vi "Dashboard Main.vi"() -> ()   [LabVIEW 2012]
uses:
  <vilib>/event_ctls.llb/eventvkey.ctl
  <vilib>/Utility/miscctls.llb/LVPointTypeDef.ctl
  <vilib>/Utility/config.llb/Read Key (String).vi
  <vilib>/Utility/config.llb/Read Key (I32).vi
  <vilib>/Utility/config.llb/Write Key (String).vi
  <vilib>/Utility/config.llb/Write Key (I32).vi
  <vilib>/Utility/config.llb/NI_LVConfig.lvlib
panel:
  out "Battery Value":dbl(slide) scale=0.0..14.0 scale format="%#_2e"
  out "Battery":sgl(graph)
  in  "Camera Settings":T1={"Frate Rate"=30, "Compression"=30, "Size"=0} {"Frate Rate" scale=1.0..30.0; "Size" items=["640x480", "320x240", "160x120"]}
  out "Mode":T2(ring)=enum.""
  out "Camera IP":string="10.16.76.11"
  out "JS1 Z":dbl(slide) scale=-1.0..1.0 scale format="%#_2e"
  out "JS2 Z":dbl(slide) scale=-1.0..1.0 scale format="%#_2e"
  out "Joystick 1":cluster{"X":dbl, "Y":dbl}[](graph)
  out "Joystick 2":cluster{"X":dbl, "Y":dbl}[](graph)
  out "JS Buttons 1":T3
  out "JS Buttons 2":T3
  out "MotorSlide4":dbl(slide) scale=-1.0..1.0 scale format="%#_2e"
  out "MotorSlide3":dbl(slide) scale=-1.0..1.0 scale format="%#_2e"
  out "MotorSlide2":dbl(slide) scale=-1.0..1.0 scale format="%#_2e"
  in  "MotorName3":string="Front Left"
  in  "MotorName4":string="Front Right"
  in  "MotorName1":string="Rear Left"
  in  "MotorName2":string="Rear Right"
  out "MotorChart4":dbl(graph)
  out "MotorChart3":dbl(graph)
  out "MotorChart2":dbl(graph)
  out "MotorSlide1":dbl(slide) scale=-1.0..1.0 scale format="%#_2e"
  out "MotorChart1":dbl(graph)
  out "Robot IP":string="0.0.0.0"
  in  "Dashboard Tab":enum32{"Operation", "Test", "Checklist"}(tab)
  out "Dashboard Code Verzion":string
  out "Robot Code Verzion":string
  out "Gyro":dbl
  out "Encoder Average":dbl
  out "Right Encoder":dbl
  out "Left Encoder":dbl
  out "Vision Angle":dbl
  out "Wheel Speed":dbl
  in  "Process Vision":bool=TRUE
  in  "Slider":dbl(slide) scale=0.0..100.0 scale format="%#_3g"
  in  "On/Off":bool caption="Solenoid"
  in  "Test Name":u16(ring) items=["Select the test to run...", "Example Test", "-------------------------------", "List of tests is built in robot code.", "Replace with your own automated tests."]
  in  "Test Tree":string(tree)
  in  "Motor":cluster{"Value":dbl, "Enable":bool} {"Value" scale=-1.0..1.0 scale format="%#_3g"}
  out "Progress":T4 {"Test Progress" scale=0.0..100.0}
  in  "Rev/Fwd":cluster{"Forward":bool, "Reverse":bool}
  in  "Ring":u16(ring) items=["Auto", "Fixed indoor", "Fixed outdoor 1", "Fixed outdoor 2", "Fixed fluorescent 1", "Fixed fluorescent 2", "Hold current"]
  in  "Listbox":i32(listbox)
  in  "Viewer":T5(tab)
  out "Mbps":dbl format="%#.1g"
  in  "Enable":bool=TRUE
  in  "DB Camera Config":bool
  out "Mbps":bool
  out "fps":dbl format="%#.1g"
  out "Image Error Message":string="Timeout in Camera Communications"
  out "Camera Image":T6(plugin-control)
  out "Buttons 1":cluster{"1":bool, "2":bool, "3":bool}
  out "Kinect 1":cluster{"X":dbl, "Y":dbl, "Z":dbl} {"X" scale=1.0..-1.0; "Y" scale=1.0..-1.0; "Z" scale=1.0..-1.0}
  out "Buttons 2":cluster{"1":bool, "2":bool, "3":bool}
  out "Kinect 2":cluster{"X":dbl, "Y":dbl, "Z":dbl} {"X" scale=1.0..-1.0; "Y" scale=1.0..-1.0; "Z" scale=1.0..-1.0}
  out "Version":string
  out "Skeleton Picture":picture
  out "Players":i8
  out "Tree":string(tree)
  # "Drive & Motors"
  # "Robot IP:"
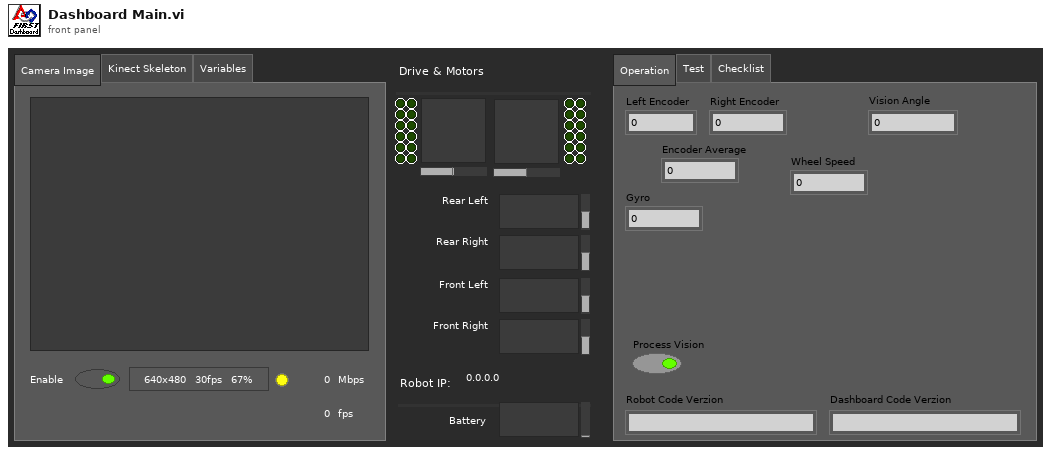
[diagram p1: front panel]
types:
  T1 = cluster{"Frate Rate":i32, "Compression":i32, "Size":u16}
  T2 = enum8{"Tele-Op Disabled", "Tele-Op Enabled", "Auto Disabled", "Auto Enabled", "Test Disabled", "Test Enabled", ""}
  T3 = cluster{bool, bool, bool, bool, bool, bool, bool, bool, bool, bool, bool, bool}
  T4 = cluster{"Test Progress":u8, "Test Progress Text":string}
  T5 = enum32{"Camera Image", "Kinect Skeleton", "Variables"}
  T6 = typedef "IMAQ Image.ctl" = refnum<image>
  T7 = typedef "Image Type" = u32
  T8 = cluster{"Competition mode":bool, "Robot Link":bool, "Autonomous":bool, "Enabled":bool, "E-Stop":bool, "Simulated":bool, "TestMode":bool, "Docked Window":bool}
  T9 = cluster{"Boolean Array[0]":bool, "Boolean Array[1]":bool, "Boolean Array[2]":bool, "Boolean Array[3]":bool, "Boolean Array[4]":bool, "Boolean Array[5]":bool, "Boolean Array[6]":bool, "Boolean Array[7]":bool, "Boolean Array[8]":bool, "Boolean Array[9]":bool, "Boolean Array[10]":bool, "Boolean Array[11]":bool}
  T10 = typedef "LVPointTypeDef.ctl" = cluster{"Horizontal":i16, "Vertical":i16}
  T11 = typedef "LVRectTypeDef.ctl" = cluster{"Left":i16, "Top":i16, "Right":i16, "Bottom":i16}
  T12 = typedef "LVBoundsTypeDef.ctl" = cluster{"Width":u32, "Height":u32}
  T13 = typedef "SkeletonTrackState.ctl" = enum32{"NotTracked", "PositionOnly", "Tracked"}
  T14 = cluster{"TrackingState":u8[], "Position":cluster{"x":sgl, "y":sgl, "z":sgl}, cluster{"x":sgl, "y":sgl, "z":sgl, sgl}[], "TrackState":T13}
  T15 = cluster{cluster{"ScaledToPercentRange":dbl, "ScaledToPercentRange":dbl, "ScaledToPercentRange":dbl}, cluster{bool, bool, bool}}[]
  T16 = cluster{cluster{"ScaledToPercentRange":dbl, "ScaledToPercentRange":dbl, "ScaledToPercentRange":dbl}, cluster{bool, bool, bool}}
  T17 = cluster{"ScaledToPercentRange":dbl, "ScaledToPercentRange":dbl, "ScaledToPercentRange":dbl}
  T18 = typedef "NI_LVConfig.lvlib/Config Data RefNum.ctl" = refnum<k1>
  T19 = typedef "eventvkey.ctl" = enum16{"ASCII", "Enter", "Return", "Shift", "Ctrl", "Alt", "Cmd", "Opt", "Caps", "NumLock", "Clear", "Break", "Up", "Down", "Left", "Right", "Insert", "Delete", "Home", "End", "PageUp", "PageDown", "Escape", "Help", "Pause", "ScrollLock", "F1", "F2", "F3", "F4", "F5", "F6", "F7", "F8", "F9", "F10", "F11", "F12", "F13", "F14", "F15", "F16", "F17", "F18", "F19", "F20", "F21", "F22", "F23", "F24", "Play", "VolumeUp", "VolumeDown", "Mute", "Two Byte Char"}
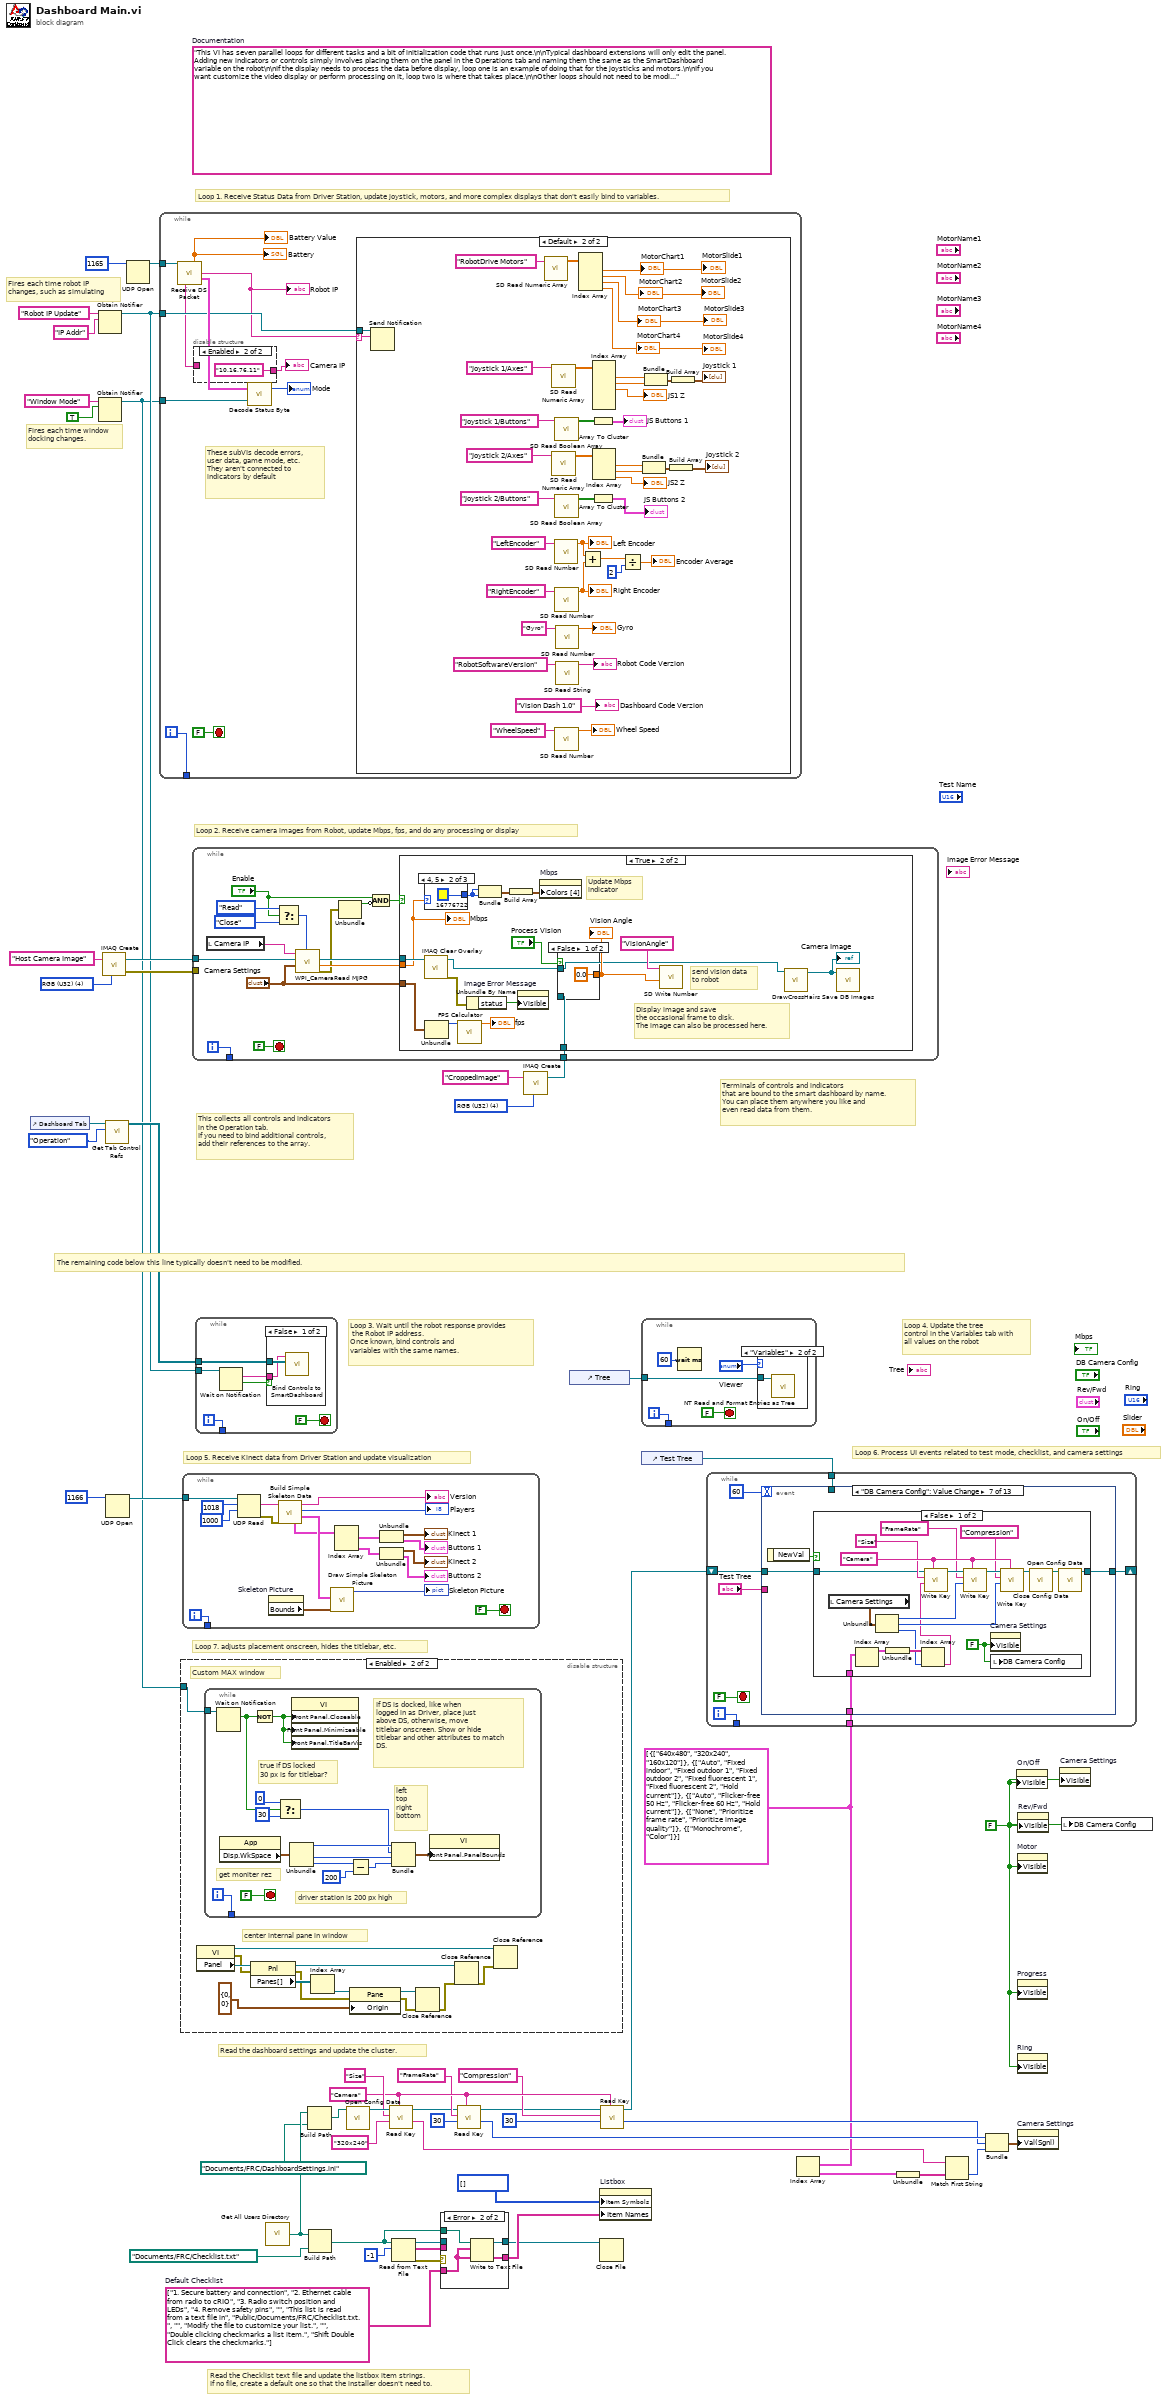
[diagram p0: block diagram]
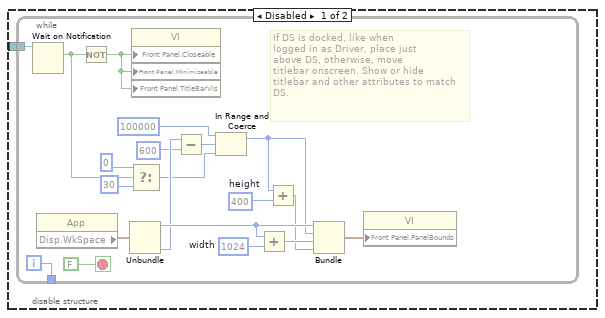
[diagram p2: hidden frame]
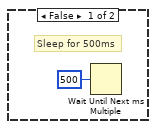
[diagram p4: hidden frame]
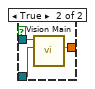
[diagram p5: hidden frame]
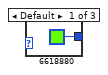
[diagram p6: hidden frame]
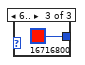
[diagram p7: hidden frame]
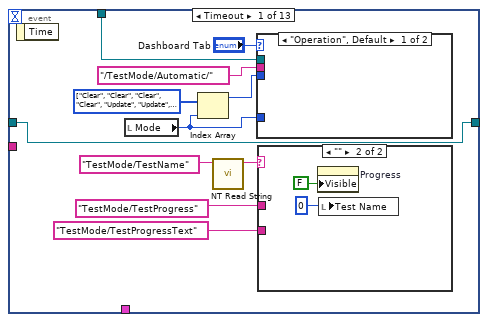
[diagram p9: hidden frame]
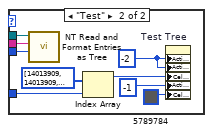
[diagram p10: hidden frame]
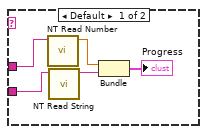
[diagram p11: hidden frame]
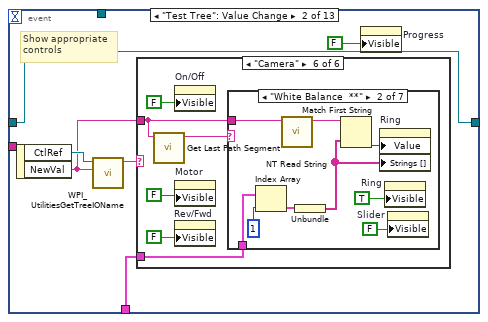
[diagram p12: hidden frame]
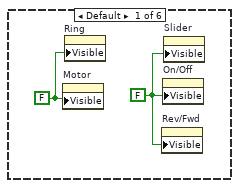
[diagram p13: hidden frame]
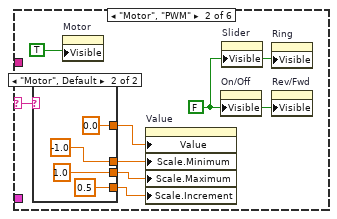
[diagram p14: hidden frame]
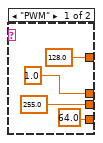
[diagram p15: hidden frame]
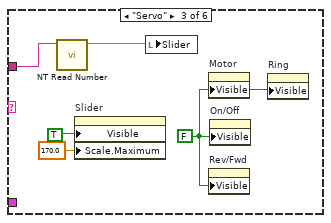
[diagram p16: hidden frame]
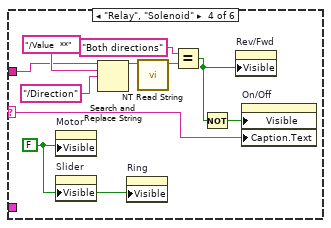
[diagram p17: hidden frame]
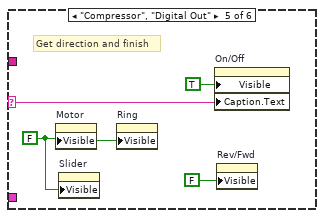
[diagram p18: hidden frame]
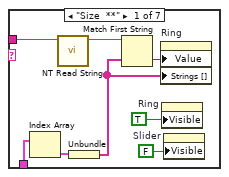
[diagram p19: hidden frame]
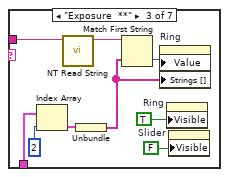
[diagram p20: hidden frame]
diagram:
  w2 = T7 4 items=["Grayscale (U8)", "Grayscale (I16)", "Grayscale (SGL)", "Complex (CSG)", "RGB (U32)", "HSL (U32)", "RGB (U64)", "Grayscale (U16)"] ("Image Type")
  w24 = "Camera"
  w16 = cluster{string[]}[] [{["640x480", "320x240", "160x120"]}, {["Auto", "Fixed indoor", "Fixed outdoor 1", "Fixed outdoor 2", "Fixed fluorescent 1", "Fixed fluorescent 2", "Hold current"]}, {["Auto", "Flicker-free 50 Hz", "Flicker-free 60 Hz", "Hold current"]}, {["None", "Prioritize frame rate", "Prioritize image quality"]}, {["Monochrome", "Color"]}]
  w32 = string[] ["1. Secure battery and connection", "2. Ethernet cable from radio to cRIO", "3. Radio switch position and LEDs", "4. Remove safety pins", "", "This list is read from a text file in", "Public/Documents/FRC/Checklist.txt.", "", "Modify the file to customize your list.", "", "Double clicking checkmarks a list item.", "Shift Double Click clears the checkmarks."]  # Default Checklist
  w30 = FALSE ("Visible")
  (unwired) "This VI has seven parallel loops for different tasks and a bit of initialization code that runs just once.\n\nTypical dashboard extensions will only edit the panel. Adding new indicators or controls simply involves placing them on the panel in the Operations tab and naming them the same as the SmartDashboard variable on the robot\n\nIf the display needs to process the data before display, loop one is an example of doing that for the joysticks and motors.\n\nIf you want customize the video display or perform processing on it, loop two is where that takes place.\n\nOther loops should not need to be modified. They are pretty standard, and document the task they perform."  # Documentation
  w53 = T7 4 items=["Grayscale (U8)", "Grayscale (I16)", "Grayscale (SGL)", "Complex (CSG)", "RGB (U32)", "HSL (U32)", "RGB (U64)"] ("Image Type")
  # "Fires each time robot IP\nchanges, such as simulating"
  # "Fires each time window\ndocking changes."
  # "Read the Checklist text file and update the listbox item strings.\nIf no file, create a default one so that the installer doesn't need to."
  # "This collects all controls and indicators\nin the Operation tab.\nIf you need to bind additional controls,\nadd their references to the array."
  # "The remaining code below this line typically doesn't need to be modified."
  # "Loop 6. Process UI events related to test mode, checklist, and camera settings"
  # "Read the dashboard settings and update the cluster."
  # "Terminals of controls and indicators\nthat are bound to the smart dashboard by name.\nYou can place them anywhere you like and\neven read data from them."
  # "Loop 4. Update the tree\ncontrol in the Variables tab with\nall values on the robot"
  # "Loop 3. Wait until the robot response provides\n the Robot IP address.\nOnce known, bind controls and\nvariables with the same names."
  # "Loop 5. Receive Kinect data from Driver Station and update visualization"
  # "Loop 7. adjusts placement onscreen, hides the titlebar, etc."
  # "Loop 1. Receive Status Data from Driver Station, update joystick, motors, and more complex displays that don't easily bind to variables."
  # "Loop 2. Receive camera images from Robot, update Mbps, fps, and do any processing or display"
  n1 = control-ref of="Dashboard Tab"() -> (w46:refnum<vi>)
  n2 = Obtain Notifier(name (unnamed)="Robot IP Update", notification data type="IP Addr" ("name (unnamed)")) -> (notifier out=w43:refnum<notifier>)  [unwired: 2 in, 2 out]
  n3 = Obtain Notifier(name (unnamed)="Window Mode", notification data type=TRUE) -> (notifier out=w36:refnum<notifier>)  [unwired: 2 in, 2 out]
  n4 = call "IMAQ Create"("Image Name"="Host Camera Image", "Image Type"=w53) -> ("New Image"=w51:T6, "error out"=w50:errorcluster)  [unwired: 2 in, 1 out]
  n5 = call <vilib>:"Get Tab Control Refs.vi"("Page Index"=enum32{"Operation", "Test"}."Operation" ("Dashboard Tab"), "TabControl in"=w46) -> ("ControlsOnPage"=w47:refnum<vi>[])  [unwired: 9 in]
  n6 = UDP Open(11:u16 1166 ("port")) -> (port=w48:refnum<k16>)  [unwired: 2 in, 4 out]
  n7 = UDP Open(11:u16 1165 ("port")) -> (port=w54:refnum<k16>)  [unwired: 2 in, 4 out]
  n8 = while {
    tunnel: w54 -> [w64]
    tunnel: w43 -> [w59]
    tunnel: w36 -> [w62]
    tunnel: [w60] -> _
    i -> [w60]
    stop <- FALSE stop-if-true
    # "These subVIs decode errors, user data, game mode, etc.\nThey aren't connected to indicators by default"
    n9 = call "Receive DS Packet.vi"("Recv Socket"=w64) -> ("Battery"=→"Battery" →"Battery Value":sgl, "Robot IP Address"=w58:string, "Status"=w65:T8, "Camera IP Address"=w56:string)  [unwired: 1 in, 10 out]
    "Robot IP" <- w58
    n10 = disable-structure shown="Enabled" {
      disable-tunnel: [w67 "10.16.76.11" ("Camera IP")] -> w57
      disable-tunnel: w56 -> [w67 _]
      frame Disabled {
      }
      frame Enabled {
      }
    }
    "Camera IP" <- w57
    n11 = call "Decode Status Byte.vi"("Window Mode Notifier"=w62, "Status"=w65) -> ("Mode"=→"Mode":T2)  [unwired: 1 out]
    n12 = case shown="Default" w58 {
      selector: w58 -> [_ w83]
      tunnel: w59 -> [_ w84]
      frame "0.0.0.0" {
        # "Robot not responding, don't poll the variables"
      }
      frame Default {
        n13 = Send Notification(notification=w83, notifier=w84) -> ()  [unwired: 1 in, 2 out]
        n14 = call <vilib>:"SD Read Numeric Array.vi"("Name"="RobotDrive Motors") -> ("Numeric Array"=w107:dbl[])  [unwired: 8 in, 2 out]
        n15 = call <vilib>:"SD Read Numeric Array.vi"("Name"="Joystick 1/Axes") -> ("Numeric Array"=w100:dbl[])  [unwired: 8 in, 2 out]
        n16 = call <vilib>:"SD Read Numeric Array.vi"("Name"="Joystick 2/Axes") -> ("Numeric Array"=w94:dbl[])  [unwired: 8 in, 2 out]
        n17 = call <vilib>:"SD Read Number.vi"("Name"="LeftEncoder") -> ("Numeric"=w79:dbl)  [unwired: 8 in, 2 out]
        "Left Encoder" <- w79
        n18 = call <vilib>:"SD Read Boolean Array.vi"("Name"="Joystick 1/Buttons") -> ("Boolean Array"=w102:bool[])  [unwired: 8 in, 2 out]
        n19 = call <vilib>:"SD Read Boolean Array.vi"("Name"="Joystick 2/Buttons") -> ("Boolean Array"=w93:bool[])  [unwired: 8 in, 2 out]
        n20 = call <vilib>:"SD Read Number.vi"("Name"="RightEncoder") -> ("Numeric"=w78:dbl)  [unwired: 8 in, 2 out]
        "Right Encoder" <- w78
        n21 = call <vilib>:"SD Read Number.vi"("Name"="WheelSpeed") -> ("Numeric"=→"Wheel Speed":dbl)  [unwired: 8 in, 2 out]
        n22 = call <vilib>:"SD Read Number.vi"("Name"="Gyro") -> ("Numeric"=→"Gyro":dbl)  [unwired: 8 in, 2 out]
        n23 = call <vilib>:"SD Read String.vi"("Name"="RobotSoftwareVersion") -> ("String"=→"Robot Code Verzion":string)  [unwired: 8 in, 2 out]
        n24 = Index Array(array=w107) -> (element #1=→"MotorChart1" →"MotorSlide1":dbl, element #2=→"MotorSlide2" →"MotorChart2":dbl, element #3=→"MotorChart3" →"MotorSlide3":dbl, element #4=→"MotorChart4" →"MotorSlide4":dbl)  [unwired: 4 in]
        n25 = Add(x=w79, y=w78) -> (x+y=w76:dbl)
        n26 = Array To Cluster(array=w102) -> (cluster=→"JS Buttons 1":T9)
        n27 = Array To Cluster(array=w93) -> (cluster=→"JS Buttons 2":T9)
        n28 = Index Array(array=w100) -> (element #1=w97:dbl, element #2=w98:dbl, element #3=→"JS1 Z":dbl)  [unwired: 6 in, 3 out]
        n29 = Index Array(array=w94) -> (element #1=w89:dbl, element #2=w88:dbl, element #3=→"JS2 Z":dbl)  [unwired: 3 in]
        n30 = Divide(x=w76, y=2) -> (x/y=→"Encoder Average":dbl)
        n31 = Bundle("Numeric"=w89, "Numeric"=w88) -> (w90:cluster{"Numeric":dbl, "Numeric":dbl})  [unwired: 1 in]
        n32 = Bundle("Numeric"=w97, "Numeric"=w98) -> (w96:cluster{"Numeric":dbl, "Numeric":dbl})  [unwired: 1 in]
        n33 = Build Array(w90) -> (→"Joystick 2":cluster{"Numeric":dbl, "Numeric":dbl}[])
        n34 = Build Array(w96) -> (→"Joystick 1":cluster{"Numeric":dbl, "Numeric":dbl}[])
        "Dashboard Code Verzion" <- "Vision Dash 1.0" ("Dashboard Code Verzion")
      }
    }
  }
  n35 = disable-structure shown="Enabled" {
    disable-tunnel: w36 -> [w111 w144]
    frame Disabled {
      n36 = while {
        tunnel: w111 -> [w130]
        tunnel: [w128] -> _
        i -> [w128]
        stop <- FALSE stop-if-true
        w120 = 1024  # width
        w123 = 400  # height
        # "If DS is docked, like when\nlogged in as Driver, place just\nabove DS, otherwise, move\ntitlebar onscreen. Show or hide\ntitlebar and other attributes to match\nDS."
        n37 = Wait on Notification(notifier=w130) -> (notification=w115:bool)  [unwired: 3 in, 3 out]
        n38 = property class="App"() -> ("Disp.WkSpace"=w126:T11)  [unwired: 2 in, 2 out]
        n39 = Not(x=w115) -> (.not. x?=w129:bool)
        n40 = Unbundle(w126) -> ("Left"=w124:i16, "Bottom"=w121:i16)  [unwired: 2 out]
        n41 = Select(t=0, s=w115, f=30) -> (s? t:f=w114:i32)
        n42 = property class="VI"("Front Panel.Closeable"=w129, "Front Panel.Minimizeable"=w129, "Front Panel.TitleBarVis"=w129) -> ()  [unwired: 2 in, 2 out]
        n43 = Subtract(x=w121, y=600) -> (x-y=w118:i32)
        n44 = In Range and Coerce(upper limit=100000, x=w118, lower limit=w114) -> (coerced(x)=w112:i32)  [unwired: 1 out]
        n45 = Add(x=w124, y=w120) -> (x+y=w125:i32)
        n46 = Add(x=w112, y=w123) -> (x+y=w122:i32)
        n47 = Bundle("Left"=w124, w112, w125, w122) -> (w127:cluster{"Left":i16, i32, i32, i32})  [unwired: 1 out]
        n48 = property class="VI"("Front Panel.PanelBounds"=w127) -> ()  [unwired: 2 in, 2 out]
      }
    }
    frame Enabled {
      # "center internal pane in window"
      # "Custom MAX window"
      n49 = property class="VI"() -> (reference out=w137:refnum<vi>, error out=w136:errorcluster, "Panel"=w143:refnum<vi>)  [unwired: 2 in]
      n50 = while {
        tunnel: w144 -> [w158]
        tunnel: [w156] -> _
        i -> [w156]
        stop <- FALSE stop-if-true
        # "driver station is 200 px high"
        # "true if DS locked\n30 px is for titlebar?"
        # "left\ntop\nright\nbottom"
        # "get moniter rez"
        # "If DS is docked, like when\nlogged in as Driver, place just\nabove DS, otherwise, move\ntitlebar onscreen. Show or hide\ntitlebar and other attributes to match\nDS."
        n51 = Wait on Notification(notifier=w158) -> (notification=w150:bool)  [unwired: 3 in, 3 out]
        n52 = property class="App"() -> ("Disp.WkSpace"=w154:T11)  [unwired: 2 in, 2 out]
        n53 = Not(x=w150) -> (.not. x?=w157:bool)
        n54 = Select(t=0, s=w150, f=30) -> (s? t:f=w148:i32)
        n55 = Unbundle(w154) -> ("Left"=w153:i16, "Right"=w149:i16, "Bottom"=w146:i16)  [unwired: 1 out]
        n56 = property class="VI"("Front Panel.Closeable"=w157, "Front Panel.Minimizeable"=w157, "Front Panel.TitleBarVis"=w157) -> ()  [unwired: 2 in, 2 out]
        n57 = Subtract(x=w146, y=i16 200) -> (x-y=w147:i16)
        n58 = Bundle("Left"=w153, w148, "Right"=w149, w147) -> (w155:cluster{"Left":i16, i32, "Right":i16, i16})  [unwired: 1 out]
        n59 = property class="VI"("Front Panel.PanelBounds"=w155) -> ()  [unwired: 2 in, 2 out]
      }
      n60 = property class="Pnl"(reference=w143, error in=w136) -> (reference out=w138:refnum<vi>, error out=w135:errorcluster, "Panes[]"=w142:refnum<vi>[])
      n61 = Index Array(array=w142) -> (element=w141:refnum<vi>)  [unwired: 1 in]
      n62 = property class="Pane"(reference=w141, error in=w135, "Origin"=T10 {"Horizontal"=0, "Vertical"=0}) -> (reference out=w139:refnum<vi>, error out=w134:errorcluster)
      n63 = Close Reference(reference=w139, error in (no error)=w134) -> (error out=w133:errorcluster)
      n64 = Close Reference(reference=w138, error in (no error)=w133) -> (error out=w132:errorcluster)
      n65 = Close Reference(reference=w137, error in (no error)=w132) -> ()  [unwired: 1 out]
    }
  }
  n66 = while {
    tunnel: w48 -> [w176]
    tunnel: [w161] -> _
    i -> [w161]
    stop <- FALSE stop-if-true
    n67 = UDP Read(connection ID=w176, max size (548)=1018 ("bytes to read"), timeout ms (25000)=1000) -> (data out=w170:string, error out=w160:errorcluster)  [unwired: 1 in, 3 out]
    n68 = property on="Skeleton Picture" class="Pict"() -> ("Bounds"=w172:T12)  [unwired: 2 in, 2 out]
    n69 = call "Build Simple Skeleton Data.vi"("error in (no error)"=w160, "data in"=w170) -> ("Skeleton Data"=w171:T14, "NumPlayers"=→"Players":i8, "Version String"=→"Version":string, "Simple Joystick Info"=w168:T15)  [unwired: 5 in, 1 out]
    n70 = call "Draw Simple Skeleton Picture.vi"("Bounds"=w172, "Simple Skeleton"=w171) -> ("new picture out"=→"Skeleton Picture":picture)  [unwired: 9 in]
    n71 = Index Array(array=w168) -> (element #1=w167:T16, element #2=w166:T16)  [unwired: 2 in]
    n72 = Unbundle(w167) -> (→"Kinect 1":T17, →"Buttons 1":cluster{bool, bool, bool})
    n73 = Unbundle(w166) -> (→"Kinect 2":T17, →"Buttons 2":cluster{bool, bool, bool})
  }
  n74 = while {
    tunnel: w47 -> [w184]
    tunnel: w43 -> [w181]
    tunnel: [w179] -> _
    i -> [w179]
    stop <- FALSE stop-if-true
    n75 = Wait on Notification(notifier=w181) -> (notification=w180:string, timed out?=w182:bool)  [unwired: 3 in, 2 out]
    n76 = case shown="False" w182 {
      tunnel: w184 -> [w186 _]
      tunnel: w180 -> [w185 _]
      frame False {
        n77 = call <vilib>:"Bind Controls to SmartDashboard.vi"("Bound Control Refs"=w186, "Server IP Address"=w185) -> ()  [unwired: 10 in]
      }
      frame True {
      }
    }
  }
  n78 = call "Get All Users Directory.vi"() -> ("All User Path"=w29:path)
  n79 = Build Path(base path=w29, name or relative path=path "Documents/FRC/DashboardSettings.ini") -> (appended path=w28:path)
  n80 = Build Path(base path=w29, name or relative path=path "Documents/FRC/Checklist.txt") -> (appended path=w33:path)
  n81 = call <vilib>:"Open Config Data.vi"("configuration file path"=w28) -> ("refnum"=w27:T18)  [unwired: 8 in, 2 out]
  n82 = call-poly <vilib>:"Read Key.vi"("section"=w24, "default value"="320x240", "key"="Size", "refnum"=w27) -> ("value"=w14:string, "refnum out"=w9:T18)  [unwired: 2 in, 4 out]
  n83 = Read from Text File(file (use dialog)=w33, count=-1 ("timeout ms (25000)")) -> (refnum out=w11:refnum<file>, text=w34:string[], error out=w35:errorcluster)  [unwired: 2 in, 1 out]
  n84 = case shown="Error" w35 {
    tunnel: w34 -> [w188 _]
    tunnel: [w188 w190] -> w31
    tunnel: w32 -> [_ w190]
    tunnel: w33 -> [_ w191]
    tunnel: [w187 w189] -> w10
    tunnel: w11 -> [w187 _]
    frame No Error {
    }
    frame Error {
      n85 = Write to Text File(file (use dialog)=w191, text=w190) -> (refnum out=w189:refnum<file>)  [unwired: 2 in, 2 out]
    }
  }
  n86 = call-poly <vilib>:"Read Key.vi"("section"=w24, "default value"=30, "key"="FrameRate", "refnum"=w9) -> ("value"=w19:i32, "refnum out"=w8:T18)  [unwired: 1 in, 5 out]
  n87 = call "IMAQ Create"("Image Name"="CroppedImage", "Image Type"=w2) -> ("New Image"=w1:T6)  [unwired: 3 in, 1 out]
  n88 = while {
    tunnel: w51 -> [w202]
    tunnel: w50 -> [_]
    tunnel: [w205] -> _
    tunnel: w1 -> [w192]
    i -> [w205]
    stop <- FALSE stop-if-true
    n89 = local read "Camera IP"() -> (w204:string)
    n90 = Select(t=enum16{"Read", "Reopen", "Close"}."Read" ("Operation"), s="Enable", f=enum16{"Read", "Reopen", "Close"}."Close" ("Operation")) -> (s? t:f=w197:enum16{"Read", "Reopen", "Close"})
    n91 = call <vilib>:"WPI_CameraRead MJPG.vi"("Operation"=w197, "Camera Settings"="Camera Settings", "Image"=w202, "address"=w204) -> ("error out"=w196:errorcluster, "Bandwidth (kbps)"=w200:dbl, "Image Out"=w201:T6)  [unwired: 5 in]
    n92 = Unbundle(w196) -> ("status"=w194:bool)  [unwired: 2 out]
    n93 = Compound Arithmetic op=AND("Enable", invert w194) -> (w193:bool)
    n94 = case shown="True" w193 {
      tunnel: "Camera Settings" -> [_ w215]
      tunnel: w201 -> [_ w218]
      tunnel: w200 -> [_ w217]
      tunnel: w192 -> [_ w209]
      frame False {
        # "Sleep for 500ms"
        n95 = Wait Until Next ms Multiple(millisecond multiple=u32 500) -> ()  [unwired: 1 out]
      }
      frame True {
        # "send vision data\nto robot"
        # "Display image and save\nthe occasional frame to disk.\nThe image can also be processed here."
        # "Update Mbps\nindicator"
        n96 = call "IMAQ Clear Overlay"("Image"=w218) -> ("error out"=w222:errorcluster, "Image Out"=w210:T6)  [unwired: 2 in, 7 out]
        n97 = case shown="4, 5" w217 {
          tunnel: [u32 6618880 ("Color Box") u32 16776722 ("Color Box") u32 16716800 ("Color Box")] -> w219
          frame Default {
          }
          frame 4, 5 {
          }
          frame 6.. {
          }
        }
        n98 = Unbundle(w215) -> ("Frate Rate"=w214:i32)  [unwired: 2 out]
        n99 = call "FPS Calculator.vi"("Average Count"=w214) -> ("fps"=→"fps":dbl)  [unwired: 10 in]
        n100 = Unbundle By Name(w222) -> ("status"=w223:bool)
        n101 = Bundle("Color Box"=w219, "Color Box"=w219) -> (w221:cluster{"Color Box":u32, "Color Box":u32})  [unwired: 1 out]
        n102 = Build Array(w221) -> (w220:cluster{"Color Box":u32, "Color Box":u32}[])
        n103 = property on="Image Error Message" class="Str"("Visible"=w223) -> ()  [unwired: 2 in, 2 out]
        n104 = property on="Mbps" class="Bool (strict)"("Colors [4]"=w220) -> ()  [unwired: 2 in, 2 out]
        n105 = case shown="False" "Process Vision" {
          tunnel: [0.0 ("Chosen Target Angle") w227] -> w212
          tunnel: w210 -> [_ w226]
          tunnel: w209 -> [_ w225]
          frame False {
          }
          frame True {
            n106 = call "Vision Main.vi"("Cropped Image"=w225, "Camera Image"=w226) -> ("Chosen Target Angle"=w227:dbl)  [unwired: 8 in, 1 out]
          }
        }
        "Vision Angle" <- w212
        n107 = call <vilib>:"SD Write Number.vi"("Numeric"=w212, "Name"="VisionAngle") -> ()  [unwired: 8 in, 2 out]
        n108 = call "DrawCrossHairs.vi"("Image In"=w210) -> ("Image Out"=w211:T6)  [unwired: 10 in]
        "Camera Image" <- w211
        n109 = call "Save DB Images.vi"("Image"=w211) -> ()  [unwired: 2 in, 1 out]
        "Mbps" <- w217
      }
    }
  }
  n110 = control-ref of="Tree"() -> (w5:refnum<vi>)
  n111 = property on="Listbox" class="LstBox (strict)"("Item Symbols"=i32[] [], "Item Names"=w31) -> ()  [unwired: 2 in, 2 out]
  n112 = Close File(refnum=w10) -> ()  [unwired: 1 in, 2 out]
  n113 = call-poly <vilib>:"Read Key.vi"("section"=w24, "default value"=30, "key"="Compression", "refnum"=w8) -> ("value"=w18:i32, "refnum out"=w6:T18)  [unwired: 1 in, 5 out]
  n114 = while {
    tunnel: [w232] -> _
    tunnel: w5 -> [w231]
    i -> [w232]
    stop <- FALSE stop-if-true
    n115 = Wait (ms)(milliseconds to wait=u32 60) -> ()  [unwired: 1 out]
    n116 = case shown="\"Variables\"" "Viewer" {
      tunnel: w231 -> [_ w236]
      frame Default {
      }
      frame "Variables" {
        n117 = call <vilib>:"NT Read and Format Entries as Tree.vi"("Tree Refnum"=w236) -> ()  [unwired: 9 in, 2 out]
      }
    }
  }
  n118 = control-ref of="Test Tree"() -> (w4:refnum<vi>)
  n119 = while {
    tunnel: w16 -> [w241]
    shift-right: [w240] -> _
    shift-left: w6 -> [w239]
    tunnel: [w238] -> _
    tunnel: w4 -> [w237]
    i -> [w238]
    stop <- FALSE stop-if-true
    n120 = event shown="[6] \"DB Camera Config\": Value Change" {
      selector: _ -> [_ _ _ _ _ _ _ _ _ _ _ _ _]
      dyn-events: _ -> [_ _ _ _ _ _ _ _ _ _ _ _ _]
      timeout: u32 60 ("milliseconds to wait") -> [_ _ _ _ _ _ _ _ _ _ _ _ _]
      tunnel: w237 -> [w251 _ _ _ _ _ _ _ _ _ _ _ _]
      tunnel: "Test Tree" -> [_ _ _ _ _ _ _ _ w445 w453 w455 w459 w467]
      tunnel: w241 -> [_ w273 _ _ _ _ w409 w439 _ _ _ _ _]
      tunnel: [w245 w272 _ w375 w383 w395 w408 w432 w444 w451 w454 w458 w466] -> w240
      tunnel: w239 -> [w245 w272 _ w375 w383 w395 w407 w432 w444 w451 w454 w458 w466]
      event Timeout {
        w250 = enum16{"Update", "Clear"}[] [enum."Clear", enum."Clear", enum."Clear", enum."Clear", enum."Update", enum."Update", enum."Clear"] items=["Update", "Clear"]
        n121 = event-data() -> ()  [unwired: 1 in, 1 out]
        n122 = local read "Mode"() -> (w248:T2)
        n123 = Index Array(array=w250, index=w248) -> (element=w249:enum16{"Update", "Clear"})
        n124 = call <vilib>:"NT Read String.vi"("Name"="TestMode/TestName") -> ("String"=w254:string)  [unwired: 9 in, 1 out]
        n125 = case shown="\"Operation\", Default" "Dashboard Tab" {
          tunnel: w251 -> [_ w264]
          tunnel: "/TestMode/Automatic/" ("Name Pattern") -> [_ w263]
          tunnel: w249 -> [_ w262]
          tunnel: w248 -> [_ w260]
          frame "Operation", Default {
          }
          frame "Test" {
            w259 = -2 ("Active Item:Row Number")
            n126 = call <vilib>:"NT Read and Format Entries as Tree.vi"("Operation"=w262, "Name Pattern"=w263, "Tree Refnum"=w264) -> ()  [unwired: 7 in, 2 out]
            n127 = Index Array(array=u32[] [14013909, 14013909, 14013909, 14013909, 14013909, 16777215, 14013909], index=w260) -> (element=w258:u32)
            n128 = property on="Test Tree" class="Tree (strict)"("Active Item Row Number"=w259, "ActiveColNum"=w259, "CellBG"=w258, "Active Item Row Number"=-1 ("Active Item:Row Number"), "CellBG"=u32 5789784 ("Color Box")) -> ()  [unwired: 2 in, 2 out]
          }
        }
        n129 = case shown="\"\"" w254 {
          tunnel: "TestMode/TestProgress" ("Name") -> [w266 _]
          tunnel: "TestMode/TestProgressText" ("Name") -> [w265 _]
          frame Default {
            n130 = call <vilib>:"NT Read Number.vi"("Name"=w266) -> ("Numeric"=w267:dbl)  [unwired: 9 in, 1 out]
            n131 = call <vilib>:"NT Read String.vi"("Name"=w265) -> ("String"=w268:string)  [unwired: 9 in, 1 out]
            n132 = Bundle("Numeric"=w267, "String"=w268) -> (→"Progress":cluster{"Numeric":dbl, "String":string})  [unwired: 1 in]
          }
          frame "" {
            n133 = property on="Progress" class="Clust (strict)"("Visible"=FALSE) -> ()  [unwired: 2 in, 2 out]
            n134 = local write "Test Name"(u16 0) -> ()
          }
        }
      }
      event "Test Tree": Value Change {
        # "Show appropriate\ncontrols"
        n135 = event-data() -> ("CtlRef"=w276:refnum<vi>, "NewVal"=w274:string)  [unwired: 1 in]
        n136 = call <vilib>:"WPI_UtilitiesGetTreeIOName.vi"("NewVal"=w274, "TreeControl in"=w276) -> ("I/O Name"=w277:string)  [unwired: 9 in]
        n137 = case shown="\"Camera\"" w277 {
          selector: w277 -> [_ w284 _ w302 w311 _]
          tunnel: w274 -> [_ _ w299 w301 _ w318]
          tunnel: w273 -> [_ _ _ _ _ w317]
          frame Default {
            w279 = FALSE ("Visible")
            w278 = FALSE ("Visible")
            n138 = property on="Motor" class="Clust (strict)"("Visible"=w278) -> ()  [unwired: 2 in, 2 out]
            n139 = property on="Ring" class="Ring (strict)"("Visible"=w278) -> ()  [unwired: 2 in, 2 out]
            n140 = property on="Rev/Fwd" class="Clust (strict)"("Visible"=w279) -> ()  [unwired: 2 in, 2 out]
            n141 = property on="On/Off" class="Bool (strict)"("Visible"=w279) -> ()  [unwired: 2 in, 2 out]
            n142 = property on="Slider" class="Slide (strict)"("Visible"=w279) -> ()  [unwired: 2 in, 2 out]
          }
          frame "Motor", "PWM" {
            w285 = FALSE ("Visible")
            n143 = case shown="\"Motor\", Default" w284 {
              tunnel: [1.0 ("Value") -1.0 ("Value")] -> w283
              tunnel: [255.0 ("Value") 1.0 ("Value")] -> w282
              tunnel: [128.0 ("Value") 0.0 ("Value")] -> w281
              tunnel: [64.0 ("Value") 0.5 ("Value")] -> w280
              frame "PWM" {
              }
              frame "Motor", Default {
              }
            }
            n144 = property on="Motor" class="Clust (strict)"("Visible"=TRUE) -> ()  [unwired: 2 in, 2 out]
            n145 = property on="Value" class="Slide (strict)"("Value"=w281, "Scale.Minimum"=w283, "Scale.Maximum"=w282, "Scale.Increment"=w280) -> ()  [unwired: 2 in, 2 out]
            n146 = property on="On/Off" class="Bool (strict)"("Visible"=w285) -> ()  [unwired: 2 in, 2 out]
            n147 = property on="Slider" class="Slide (strict)"("Visible"=w285) -> ()  [unwired: 2 in, 2 out]
            n148 = property on="Ring" class="Ring (strict)"("Visible"=w285) -> ()  [unwired: 2 in, 2 out]
            n149 = property on="Rev/Fwd" class="Clust (strict)"("Visible"=w285) -> ()  [unwired: 2 in, 2 out]
          }
          frame "Servo" {
            w297 = FALSE ("Visible")
            n150 = call <vilib>:"NT Read Number.vi"("Name"=w299) -> ("Numeric"=w298:dbl)  [unwired: 9 in, 1 out]
            n151 = property on="Slider" class="Slide (strict)"("Visible"=TRUE, "Scale.Maximum"=170.0 ("Scale.Range:Maximum")) -> ()  [unwired: 2 in, 2 out]
            n152 = local write "Slider"(w298) -> ()
            n153 = property on="Motor" class="Clust (strict)"("Visible"=w297) -> ()  [unwired: 2 in, 2 out]
            n154 = property on="Rev/Fwd" class="Clust (strict)"("Visible"=w297) -> ()  [unwired: 2 in, 2 out]
            n155 = property on="On/Off" class="Bool (strict)"("Visible"=w297) -> ()  [unwired: 2 in, 2 out]
            n156 = property on="Ring" class="Ring (strict)"("Visible"=w297) -> ()  [unwired: 2 in, 2 out]
          }
          frame "Relay", "Solenoid" {
            w300 = FALSE ("Visible")
            n157 = property on="Motor" class="Clust (strict)"("Visible"=w300) -> ()  [unwired: 2 in, 2 out]
            n158 = property on="Slider" class="Slide (strict)"("Visible"=w300) -> ()  [unwired: 2 in, 2 out]
            n159 = Search and Replace String(input string=w301, search string="/Value  **", replace string="/Direction") -> (result string=w307:string)  [unwired: 5 in, 3 out]
            n160 = property on="Ring" class="Ring (strict)"("Visible"=w300) -> ()  [unwired: 2 in, 2 out]
            n161 = call <vilib>:"NT Read String.vi"("Name"=w307) -> ("String"=w305:string)  [unwired: 9 in, 1 out]
            n162 = Equal?(x="Both directions", y=w305) -> (x = y?=w303:bool)
            n163 = Not(x=w303) -> (.not. x?=w304:bool)
            n164 = property on="Rev/Fwd" class="Clust (strict)"("Visible"=w303) -> ()  [unwired: 2 in, 2 out]
            n165 = property on="On/Off" class="Bool (strict)"("Visible"=w304, "Caption.Text"=w302) -> ()  [unwired: 2 in, 2 out]
          }
          frame "Compressor", "Digital Out" {
            w310 = FALSE ("Visible")
            # "Get direction and finish"
            n166 = property on="Motor" class="Clust (strict)"("Visible"=w310) -> ()  [unwired: 2 in, 2 out]
            n167 = property on="Slider" class="Slide (strict)"("Visible"=w310) -> ()  [unwired: 2 in, 2 out]
            n168 = property on="Ring" class="Ring (strict)"("Visible"=w310) -> ()  [unwired: 2 in, 2 out]
            n169 = property on="On/Off" class="Bool (strict)"("Visible"=TRUE, "Caption.Text"=w311) -> ()  [unwired: 2 in, 2 out]
            n170 = property on="Rev/Fwd" class="Clust (strict)"("Visible"=FALSE) -> ()  [unwired: 2 in, 2 out]
          }
          frame "Camera" {
            n171 = call <vilib>:"Get Last Path Segment.vi"("String in"=w318) -> ("String out"=w319:string)  [unwired: 10 in]
            n172 = property on="On/Off" class="Bool (strict)"("Visible"=FALSE) -> ()  [unwired: 2 in, 2 out]
            n173 = property on="Motor" class="Clust (strict)"("Visible"=FALSE) -> ()  [unwired: 2 in, 2 out]
            n174 = property on="Rev/Fwd" class="Clust (strict)"("Visible"=FALSE) -> ()  [unwired: 2 in, 2 out]
            n175 = case shown="\"White Balance  **\"" w319 {
              tunnel: w318 -> [w325 w334 w343 w352 w361 _ w367]
              tunnel: w317 -> [w323 w331 w340 w349 w358 _ _]
              frame "Size  **" {
                n176 = Index Array(array=w323) -> (element=w322:cluster{string[]})  [unwired: 1 in]
                n177 = call <vilib>:"NT Read String.vi"("Name"=w325) -> ("String"=w324:string)  [unwired: 9 in, 1 out]
                n178 = Unbundle(w322) -> (w320:string[])
                n179 = Match First String(2:w320, 3:w324) -> (0:w321:i32)  [unwired: 1 out]
                n180 = property on="Ring" class="Ring (strict)"("Value"=w321, "Strings []"=w320) -> ()  [unwired: 2 in, 2 out]
                n181 = property on="Ring" class="Ring (strict)"("Visible"=TRUE) -> ()  [unwired: 2 in, 2 out]
                n182 = property on="Slider" class="Slide (strict)"("Visible"=FALSE) -> ()  [unwired: 2 in, 2 out]
              }
              frame "White Balance  **" {
                n183 = Index Array(array=w331, index=1) -> (element=w332:cluster{string[]})
                n184 = call <vilib>:"NT Read String.vi"("Name"=w334) -> ("String"=w333:string)  [unwired: 9 in, 1 out]
                n185 = Unbundle(w332) -> (w329:string[])
                n186 = Match First String(2:w329, 3:w333) -> (0:w328:i32)  [unwired: 1 out]
                n187 = property on="Ring" class="Ring (strict)"("Value"=w328, "Strings []"=w329) -> ()  [unwired: 2 in, 2 out]
                n188 = property on="Ring" class="Ring (strict)"("Visible"=TRUE) -> ()  [unwired: 2 in, 2 out]
                n189 = property on="Slider" class="Slide (strict)"("Visible"=FALSE) -> ()  [unwired: 2 in, 2 out]
              }
              frame "Exposure  **" {
                n190 = Index Array(array=w340, index=2) -> (element=w341:cluster{string[]})
                n191 = call <vilib>:"NT Read String.vi"("Name"=w343) -> ("String"=w342:string)  [unwired: 9 in, 1 out]
                n192 = Unbundle(w341) -> (w337:string[])
                n193 = Match First String(2:w337, 3:w342) -> (0:w338:i32)  [unwired: 1 out]
                n194 = property on="Ring" class="Ring (strict)"("Value"=w338, "Strings []"=w337) -> ()  [unwired: 2 in, 2 out]
                n195 = property on="Ring" class="Ring (strict)"("Visible"=TRUE) -> ()  [unwired: 2 in, 2 out]
                n196 = property on="Slider" class="Slide (strict)"("Visible"=FALSE) -> ()  [unwired: 2 in, 2 out]
              }
              frame "Exposure Priority  **" {
                n197 = Index Array(array=w349, index=3) -> (element=w350:cluster{string[]})
                n198 = call <vilib>:"NT Read String.vi"("Name"=w352) -> ("String"=w351:string)  [unwired: 9 in, 1 out]
                n199 = Unbundle(w350) -> (w346:string[])
                n200 = Match First String(2:w346, 3:w351) -> (0:w347:i32)  [unwired: 1 out]
                n201 = property on="Ring" class="Ring (strict)"("Value"=w347, "Strings []"=w346) -> ()  [unwired: 2 in, 2 out]
                n202 = property on="Ring" class="Ring (strict)"("Visible"=TRUE) -> ()  [unwired: 2 in, 2 out]
                n203 = property on="Slider" class="Slide (strict)"("Visible"=FALSE) -> ()  [unwired: 2 in, 2 out]
              }
              frame "Color Enable  **" {
                n204 = Index Array(array=w358, index=4) -> (element=w359:cluster{string[]})
                n205 = call <vilib>:"NT Read String.vi"("Name"=w361) -> ("String"=w360:string)  [unwired: 9 in, 1 out]
                n206 = Unbundle(w359) -> (w355:string[])
                n207 = Match First String(2:w355, 3:w360) -> (0:w356:i32)  [unwired: 1 out]
                n208 = property on="Ring" class="Ring (strict)"("Value"=w356, "Strings []"=w355) -> ()  [unwired: 2 in, 2 out]
                n209 = property on="Ring" class="Ring (strict)"("Visible"=TRUE) -> ()  [unwired: 2 in, 2 out]
                n210 = property on="Slider" class="Slide (strict)"("Visible"=FALSE) -> ()  [unwired: 2 in, 2 out]
              }
              frame Default {
                n211 = property on="Ring" class="Ring (strict)"("Visible"=FALSE) -> ()  [unwired: 2 in, 2 out]
                n212 = property on="Slider" class="Slide (strict)"("Visible"=FALSE) -> ()  [unwired: 2 in, 2 out]
              }
              frame "Brightness  **", "Color Level  **", "Compression  **", "FPS  **", "Sharpness  **" {
                n213 = call <vilib>:"NT Read Number.vi"("Name"=w367) -> ("Numeric"=w366:dbl)  [unwired: 9 in, 1 out]
                n214 = local write "Slider"(w366) -> ()
                n215 = property on="Slider" class="Slide (strict)"("Visible"=TRUE, "Scale.Maximum"=100.0 ("Scale.Range:Maximum")) -> ()  [unwired: 2 in, 2 out]
                n216 = property on="Ring" class="Ring (strict)"("Visible"=FALSE) -> ()  [unwired: 2 in, 2 out]
              }
            }
          }
        }
        n217 = property on="Progress" class="Clust (strict)"("Visible"=FALSE) -> ()  [unwired: 2 in, 2 out]
      }
      event "Test Name": Mouse Enter {
        # "Populate the ring with the list of tests"
        n218 = event-data() -> ()  [unwired: 1 in, 1 out]
        n219 = call <vilib>:"NT Read String Array.vi"("Name"="TestMode/TestList") -> ("String Array"=w374:string[])  [unwired: 9 in, 1 out]
        n220 = Build Array (concatenate)("Select the test to run...", w374) -> (w373:string[])
        n221 = property on="Test Name" class="Ring (strict)"("Strings []"=w373) -> ()  [unwired: 2 in, 2 out]
      }
      event "Test Name": Value Change {
        w376 = FALSE ("Visible")
        # "Tell the robot the test name to run"
        n222 = event-data() -> ("NewVal"=w380:u16)  [unwired: 1 in]
        n223 = property on="Test Name" class="Ring (strict)"() -> ("Strings []"=w381:string[])  [unwired: 2 in, 2 out]
        n224 = local write "Progress"(T4 {"Test Progress"=0, "Test Progress Text"=""} ("Progress")) -> ()
        n225 = Index Array(array=w381, index=w380) -> (element=w379:string)
        n226 = call <vilib>:"NT Write String.vi"("String"=w379, "Name"="TestMode/TestName") -> ()  [unwired: 9 in, 1 out]
        n227 = property on="Progress" class="Clust (strict)"("Visible"=TRUE) -> ()  [unwired: 2 in, 2 out]
        n228 = property on="Motor" class="Clust (strict)"("Visible"=w376) -> ()  [unwired: 2 in, 2 out]
        n229 = property on="Slider" class="Slide (strict)"("Visible"=w376) -> ()  [unwired: 2 in, 2 out]
        n230 = property on="On/Off" class="Bool (strict)"("Visible"=w376) -> ()  [unwired: 2 in, 2 out]
        n231 = property on="Rev/Fwd" class="Clust (strict)"("Visible"=w376) -> ()  [unwired: 2 in, 2 out]
        n232 = property on="Ring" class="Ring (strict)"("Visible"=w376) -> ()  [unwired: 2 in, 2 out]
      }
      event "Listbox": Double Click {
        n233 = event-data() -> ("PlatMods.Shift"=w384:bool, "Row"=w386:i32)  [unwired: 1 in]
        n234 = case shown="False" w384 {
          tunnel: w386 -> [w390 _]
          tunnel: 1 -> [w389 _]
          frame False {
            n235 = property on="Listbox" class="LstBox (strict)"() -> ("Item Symbols"=w388:i32[])  [unwired: 2 in, 2 out]
            n236 = Replace Array Subset(array=w388, new element=w389, index=w390) -> (w387:i32[])
            n237 = property on="Listbox" class="LstBox (strict)"("Item Symbols"=w387) -> ()  [unwired: 2 in, 2 out]
          }
          frame True {
            w391 = 0 ("Top Row")
            n238 = property on="Listbox" class="LstBox (strict)"() -> ("Number of Rows"=w393:u32)  [unwired: 2 in, 2 out]
            n239 = Initialize Array(0, w393) -> (w392:i32[])
            n240 = property on="Listbox" class="LstBox (strict)"("Top Row"=w391, "Value"=w391, "Item Symbols"=w392) -> ()  [unwired: 2 in, 2 out]
          }
        }
      }
      event "Listbox": Key Down {
        n241 = event-data() -> ("VKey"=w397:T19)  [unwired: 1 in]
        n242 = case shown="\"Left\", \"Right\"" w397 {
          selector: w397 -> [w402 _]
          tunnel: eventvkey."Left" ("VKey") -> [w400 _]
          frame "Left", "Right" {
            n243 = Equal?(x=w400, y=w402) -> (x = y?=w401:bool)
            n244 = Select(t=0, s=w401, f=1) -> (s? t:f=w403:i32)
            n245 = property on="Listbox" class="LstBox (strict)"() -> ("Item Symbols"=w406:i32[])  [unwired: 2 in, 2 out]
            n246 = Replace Array Subset(array=w406, new element=w403, index="Listbox") -> (w405:i32[])
            n247 = property on="Listbox" class="LstBox (strict)"("Item Symbols"=w405) -> ()  [unwired: 2 in, 2 out]
          }
          frame Default {
          }
        }
      }
      event "DB Camera Config": Value Change {
        n248 = event-data() -> ("NewVal"=w410:bool)  [unwired: 1 in]
        n249 = case shown="False" w410 {
          tunnel: w409 -> [w419 _]
          tunnel: [w412 w430] -> w408
          tunnel: w407 -> [w411 w430]
          frame False {
            w426 = "Camera"
            w429 = FALSE ("Visible")
            n250 = local read "Camera Settings"() -> (w418:T1)
            n251 = Index Array(array=w419) -> (element=w422:cluster{string[]})  [unwired: 1 in]
            n252 = Unbundle(w418) -> ("Frate Rate"=w417:i32, "Compression"=w416:i32, "Size"=w420:u16)
            n253 = Unbundle(w422) -> (w421:string[])
            n254 = Index Array(array=w421, index=w420) -> (element=w415:string)
            n255 = call-poly <vilib>:"Write Key.vi"("section"=w426, "value"=w415, "key"="Size", "refnum"=w411) -> ("refnum out"=w428:T18)  [unwired: 2 in, 5 out]
            n256 = call-poly <vilib>:"Write Key.vi"("section"=w426, "value"=w417, "key"="FrameRate", "refnum"=w428) -> ("refnum out"=w427:T18)  [unwired: 1 in, 6 out]
            n257 = property on="Camera Settings" class="Clust (strict)"("Visible"=w429) -> ()  [unwired: 2 in, 2 out]
            n258 = local write "DB Camera Config"(w429) -> ()
            n259 = call-poly <vilib>:"Write Key.vi"("section"=w426, "value"=w416, "key"="Compression", "refnum"=w427) -> ("refnum out"=w413:T18)  [unwired: 1 in, 6 out]
            n260 = call <vilib>:"Close Config Data.vi"("refnum"=w413) -> ("file path"=w414:path)  [unwired: 2 in, 8 out]
            n261 = call <vilib>:"Open Config Data.vi"("configuration file path"=w414) -> ("refnum"=w412:T18)  [unwired: 8 in, 2 out]
          }
          frame True {
            n262 = property on="Camera Settings" class="Clust (strict)"("Visible"=TRUE) -> ()  [unwired: 2 in, 2 out]
          }
        }
      }
      event "Camera Settings": Value Change {
        n263 = event-data() -> ("NewVal"=w443:T1)  [unwired: 1 in]
        n264 = Index Array(array=w439) -> (element=w438:cluster{string[]})  [unwired: 1 in]
        n265 = Unbundle(w443) -> ("Frate Rate"=w434:i32, "Compression"=w433:i32, "Size"=w436:u16)
        n266 = Unbundle(w438) -> (w437:string[])
        n267 = Index Array(array=w437, index=w436) -> (element=w435:string)
        n268 = Format Into String(format string="%s   %dfps   %d%%", w435, w434, w433) -> (resulting string=w440:string)  [unwired: 2 in, 1 out]
        n269 = Build Array(w440) -> (w441:string[])
        n270 = property on="DB Camera Config" class="Bool (strict)"("Strings [4]"=w441) -> ()  [unwired: 2 in, 2 out]
      }
      event "Motor.Enable": Value Change {
        n271 = event-data() -> ("NewVal"=w449:bool)  [unwired: 1 in]
        n272 = Unbundle("Motor") -> ("Value"=w448:dbl)  [unwired: 1 out]
        n273 = Select(t=w448, s=w449, f=0.0) -> (s? t:f=w446:dbl)
        n274 = call <vilib>:"NT Write Number.vi"("Numeric"=w446, "Name"=w445) -> ()  [unwired: 9 in, 1 out]
      }
      event "Slider": Value Change {
        n275 = event-data() -> ("NewVal"=w452:dbl)  [unwired: 1 in]
        n276 = call <vilib>:"NT Write Number.vi"("Numeric"=w452, "Name"=w453) -> ()  [unwired: 9 in, 1 out]
      }
      event "On/Off": Value Change {
        n277 = event-data() -> ("NewVal"=w457:bool)  [unwired: 1 in]
        n278 = Boolean To (0,1)(Boolean=w457) -> (0, 1=w456:i16)
        n279 = call <vilib>:"NT Write Number.vi"("Numeric"=w456, "Name"=w455) -> ()  [unwired: 9 in, 1 out]
      }
      event "Rev/Fwd": Value Change {
        n280 = event-data() -> ("NewVal.Forward"=w465:bool, "NewVal.Reverse"=w464:bool)  [unwired: 1 in]
        n281 = Boolean To (0,1)(Boolean=w465) -> (0, 1=w461:i16)
        n282 = Boolean To (0,1)(Boolean=w464) -> (0, 1=w463:i16)
        n283 = Negate(x=w463) -> (-x=w462:i16)
        n284 = Add(x=w461, y=w462) -> (x+y=w460:i16)
        n285 = call <vilib>:"NT Write Number.vi"("Numeric"=w460, "Name"=w459) -> ()  [unwired: 9 in, 1 out]
      }
      event "Ring": Value Change {
        n286 = event-data() -> ("NewVal"=w469:u16)  [unwired: 1 in]
        n287 = property on="Ring" class="Ring (strict)"() -> ("Strings []"=w470:string[])  [unwired: 2 in, 2 out]
        n288 = Index Array(array=w470, index=w469) -> (element=w468:string)
        n289 = call <vilib>:"NT Write String.vi"("String"=w468, "Name"=w467) -> ()  [unwired: 9 in, 1 out]
      }
    }
  }
  n290 = Index Array(array=w16) -> (element=w17:cluster{string[]})  [unwired: 1 in]
  n291 = Unbundle(w17) -> (w15:string[])
  n292 = Match First String(2:w15, 3:w14) -> (0:w13:i32)  [unwired: 1 out]
  n293 = Bundle("value"=w19, "value"=w18, "index"=w13) -> (w7:cluster{"value":i32, "value":i32, "index":i32})  [unwired: 1 out]
  n294 = property on="On/Off" class="Bool (strict)"("Visible"=w30) -> ()  [unwired: 2 in, 2 out]
  n295 = property on="Motor" class="Clust (strict)"("Visible"=w30) -> ()  [unwired: 2 in, 2 out]
  n296 = property on="Progress" class="Clust (strict)"("Visible"=w30) -> ()  [unwired: 2 in, 2 out]
  n297 = property on="Ring" class="Ring (strict)"("Visible"=w30) -> ()  [unwired: 2 in, 2 out]
  n298 = property on="Camera Settings" class="Clust (strict)"("Val(Sgnl)"=w7) -> ()  [unwired: 2 in, 2 out]
  n299 = property on="Rev/Fwd" class="Clust (strict)"("Visible"=w30) -> ()  [unwired: 2 in, 2 out]
  n300 = property on="Camera Settings" class="Clust (strict)"("Visible"=w30) -> ()  [unwired: 2 in, 2 out]
  n301 = local write "DB Camera Config"(w30) -> ()
